vi "Dig Temp - Send Message.vi"(4 "Clock Wire Refs":refnum<vi>[](array[refnum]), 6 "SDA Refs":refnum<vi>[](array[refnum]), 7 "State":enum16{"Init", "Send", "Respond"}(ring), 8 "error in (no error)":errorcluster, 10 "Device Select":i32, 11 "t (0-100)":dbl) -> (0 "error out":errorcluster)   [LabVIEW 2014]
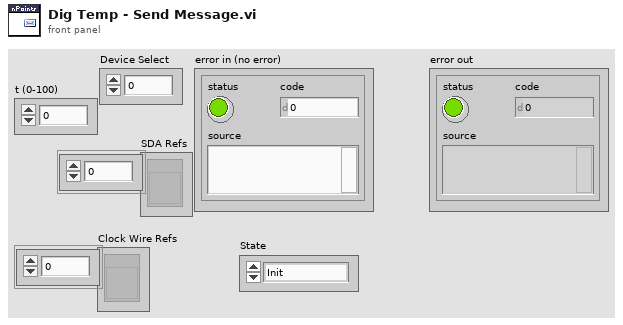
[diagram p1: front panel]
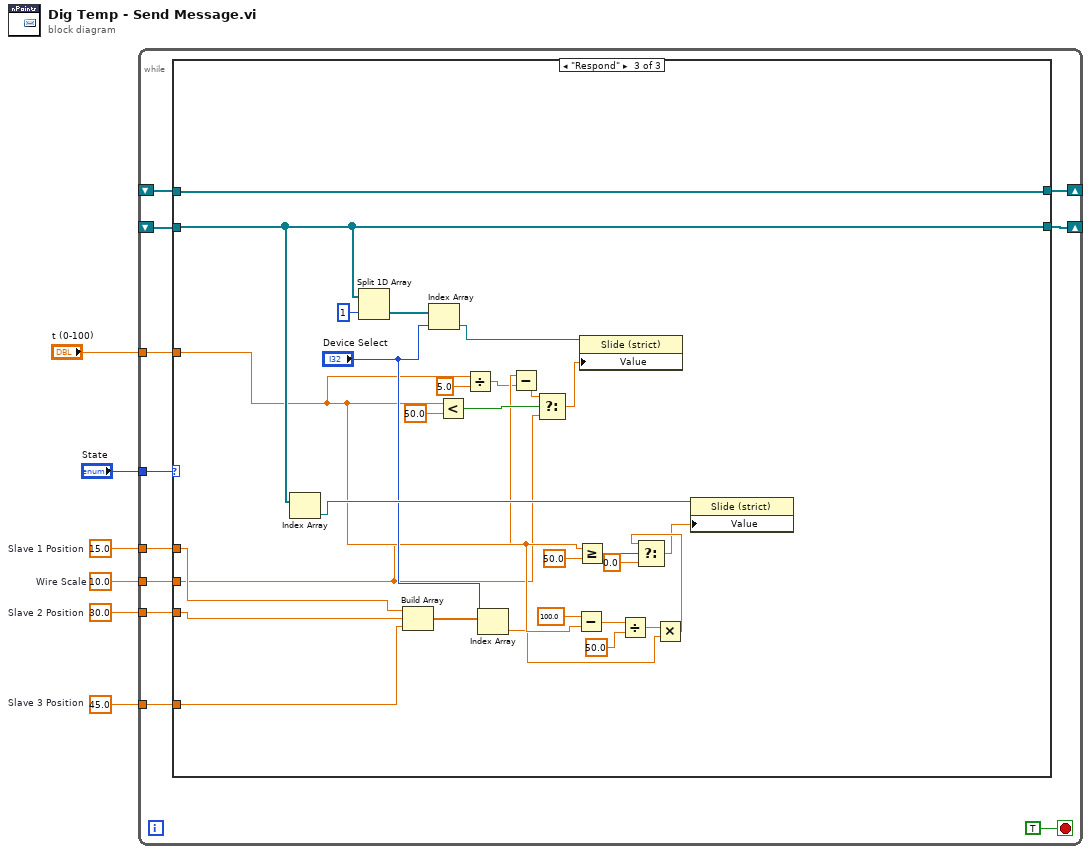
[diagram p0: block diagram]
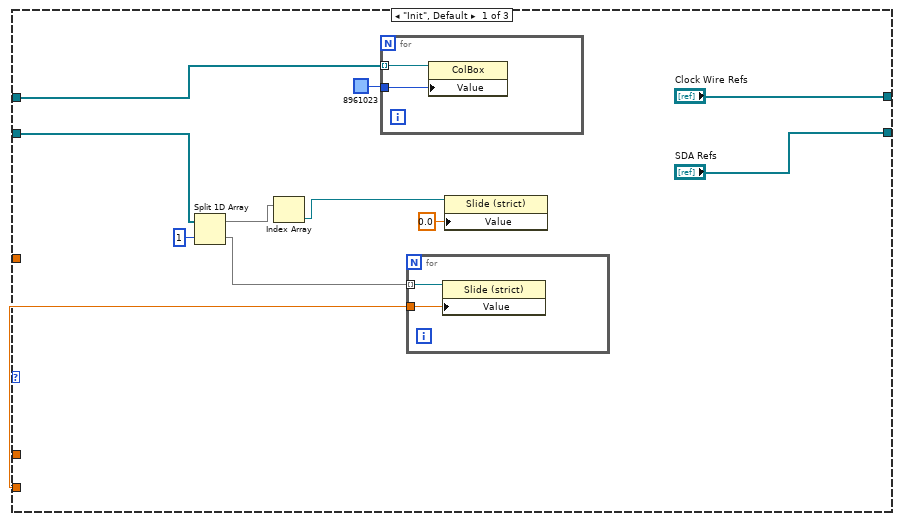
[diagram p2: hidden frame]
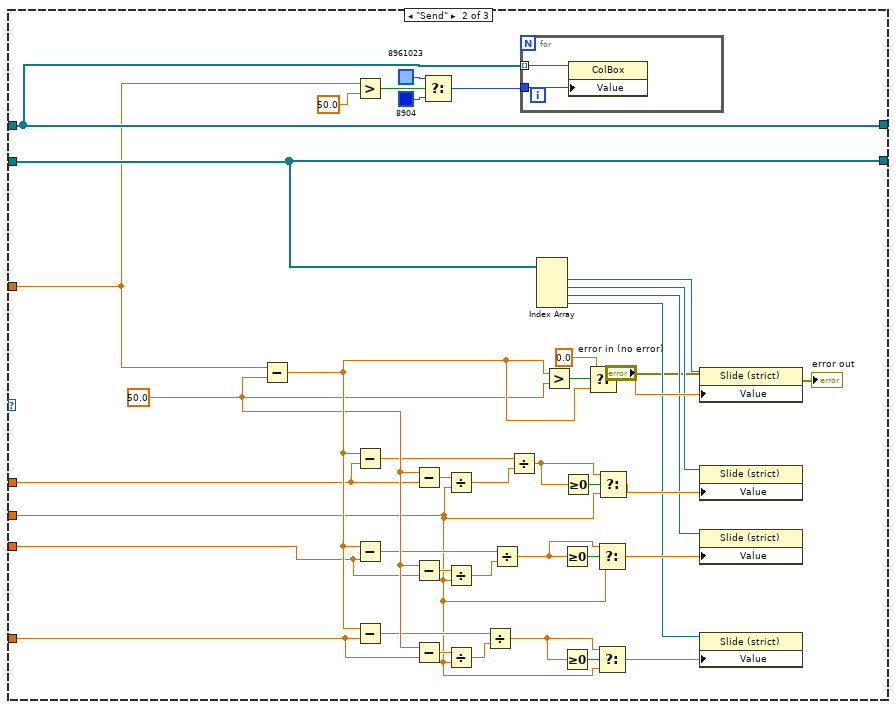
[diagram p3: hidden frame]
diagram:
  w2 = 45.0  # Slave 3 Position
  w3 = 30.0  # Slave 2 Position
  w4 = 15.0  # Slave 1 Position
  w5 = 10.0  # Wire Scale
  n1 = while {
    tunnel: "State" -> [w17]
    tunnel: w5 -> [w16]
    shift-right: [w14] -> _
    shift-left: _ -> [w13]
    shift-right: [w12] -> _
    shift-left: _ -> [w11]
    tunnel: w4 -> [w10]
    tunnel: w3 -> [w9]
    tunnel: w2 -> [w8]
    tunnel: "t (0-100)" -> [w7]
    stop <- TRUE stop-if-true
    n2 = case shown="\"Respond\"" w17 {
      tunnel: w13 -> [w27 w38 w104]
      tunnel: w11 -> [w26 w37 w96]
      tunnel: w16 -> [w23 w39 w78]
      tunnel: ["Clock Wire Refs" w38 w104] -> w14
      tunnel: ["SDA Refs" w37 w96] -> w12
      tunnel: w10 -> [_ w36 w94]
      tunnel: w9 -> [_ w35 w93]
      tunnel: w8 -> [_ w34 w92]
      tunnel: w7 -> [_ w33 w85]
      frame "Init", Default {
        n3 = Split 1D Array(array=w26, index=1) -> (first subarray=w22:refnum<vi>[], second subarray=w24:refnum<vi>[])
        n4 = Index Array(array=w22) -> (element=w21:refnum<vi>)  [unwired: 1 in]
        n5 = for {
          tunnel: w27 -> [w32] mode=indexing
          tunnel: u32 8961023 -> [w31]
          n6 = property on="Property Node" class="ColBox"(reference=w32, "Value"=w31) -> ()  [unwired: 1 in, 2 out]
        }
        n7 = for {
          tunnel: w24 -> [w30] mode=indexing
          tunnel: w23 -> [w29]
          n8 = property on="Property Node" class="Slide (strict)"(reference=w30, "Value"=w29) -> ()  [unwired: 1 in, 2 out]
        }
        n9 = property on="Property Node" class="Slide (strict)"(reference=w21, "Value"=0.0) -> ()  [unwired: 1 in, 2 out]
      }
      frame "Send" {
        w65 = 50.0 ("y")
        n10 = Subtract(x=w33, y=w65) -> (x-y=w68:dbl)
        n11 = Greater?(x=w33, y=50.0) -> (0:w47:bool)
        n12 = Subtract(x=w68, y=w36) -> (x-y=w51:dbl)
        n13 = Subtract(x=w68, y=w35) -> (x-y=w59:dbl)
        n14 = Subtract(x=w68, y=w34) -> (x-y=w60:dbl)
        n15 = Subtract(x=w65, y=w36) -> (x-y=w54:dbl)
        n16 = Subtract(x=w65, y=w35) -> (x-y=w58:dbl)
        n17 = Subtract(x=w65, y=w34) -> (x-y=w61:dbl)
        n18 = Select(t=u32 8961023, s=w47, f=u32 8904) -> (s? t:f=w73:u32)
        n19 = Divide(x=w54, y=w39) -> (x/y=w55:dbl)
        n20 = Divide(x=w58, y=w39) -> (x/y=w57:dbl)
        n21 = Divide(x=w61, y=w39) -> (x/y=w62:dbl)
        n22 = Divide(x=w60, y=w62) -> (x/y=w64:dbl)
        n23 = Divide(x=w59, y=w57) -> (x/y=w63:dbl)
        n24 = Divide(x=w51, y=w55) -> (x/y=w56:dbl)
        n25 = for {
          tunnel: w38 -> [w75] mode=indexing
          tunnel: w73 -> [w74]
          n26 = property on="Property Node" class="ColBox"(reference=w75, "Value"=w74) -> ()  [unwired: 1 in, 2 out]
        }
        n27 = Index Array(array=w37) -> (element #1=w45:refnum<vi>, element #2=w44:refnum<vi>, element #3=w43:refnum<vi>, element #4=w42:refnum<vi>)  [unwired: 4 in]
        n28 = Greater?(x=w68, y=w65) -> (0:w66:bool)
        n29 = Greater Or Equal To 0?(x=w63) -> (x >= 0?=w52:bool)
        n30 = Greater Or Equal To 0?(x=w64) -> (x >= 0?=w53:bool)
        n31 = Greater Or Equal To 0?(x=w56) -> (x >= 0?=w46:bool)
        n32 = Select(t=0.0, s=w66, f=w68) -> (s? t:f=w69:dbl)
        n33 = Select(t=w63, s=w52, f=w39) -> (s? t:f=w71:dbl)
        n34 = Select(t=w64, s=w53, f=w39) -> (s? t:f=w72:dbl)
        n35 = Select(t=w56, s=w46, f=w39) -> (s? t:f=w70:dbl)
        n36 = property on="Property Node" class="Slide (strict)"(reference=w45, error in="error in (no error)", "Value"=w69) -> (error out=→"error out":errorcluster)  [unwired: 1 out]
        n37 = property on="Property Node" class="Slide (strict)"(reference=w44, "Value"=w70) -> ()  [unwired: 1 in, 2 out]
        n38 = property on="Property Node" class="Slide (strict)"(reference=w43, "Value"=w71) -> ()  [unwired: 1 in, 2 out]
        n39 = property on="Property Node" class="Slide (strict)"(reference=w42, "Value"=w72) -> ()  [unwired: 1 in, 2 out]
      }
      frame "Respond" {
        n40 = Index Array(array=w96) -> (element=w95:refnum<vi>)  [unwired: 1 in]
        n41 = Split 1D Array(array=w96, index=1) -> (second subarray=w102:refnum<vi>[])  [unwired: 1 out]
        n42 = Build Array(w94, w93, w92) -> (w90:dbl[])
        n43 = Index Array(array=w102, index="Device Select") -> (element=w101:refnum<vi>)
        n44 = Less?(x=w85, y=50.0) -> (x < y?=w99:bool)
        n45 = Divide(x=w85, y=5.0) -> (x/y=w77:dbl)
        n46 = Index Array(array=w90, index="Device Select") -> (element=w81:dbl)
        n47 = Subtract(x=w78, y=w77) -> (x-y=w76:dbl)
        n48 = Select(t=w76, s=w99, f=w78) -> (s? t:f=w97:dbl)
        n49 = Subtract(x=100.0 ("y"), y=w85) -> (x-y=w84:dbl)
        n50 = Greater Or Equal?(x=w85, y=50.0) -> (x >= y?=w89:bool)
        n51 = property on="Property Node" class="Slide (strict)"(reference=w101, "Value"=w97) -> ()  [unwired: 1 in, 2 out]
        n52 = Divide(x=w84, y=50.0) -> (x/y=w82:dbl)
        n53 = Multiply(x=w82, y=w81) -> (x*y=w80:dbl)
        n54 = Select(t=w80, s=w89, f=0.0) -> (s? t:f=w79:dbl)
        n55 = property on="Property Node" class="Slide (strict)"(reference=w95, "Value"=w79) -> ()  [unwired: 1 in, 2 out]
      }
    }
  }
